vi "Unflatten-JoyButtonEventData.vi"(8 "error in (no error)":errorcluster, 11 "Event Binary Data":string) -> (0 "error out":errorcluster, 3 "Event Data":T1)   [LabVIEW 2026, in "SDL3.lvlib" / "Events.lvlib"]
uses:
  JoyButtonEventData--cluster.ctl
  Joystick/JoystickID--integer.ctl
  Events.lvlib
  Joystick/Joystick.lvlib
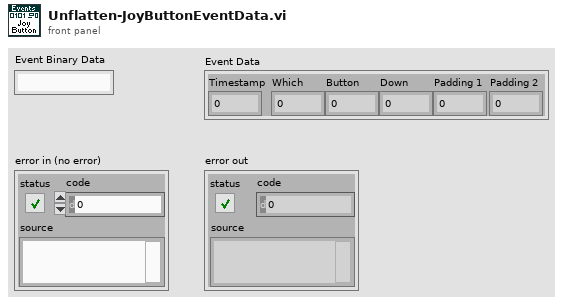
[diagram p1: front panel]
types:
  T1 = typedef "SDL3.lvlib/Events.lvlib/JoyButtonEventData--cluster.ctl" = cluster{"Timestamp":u64, "Which":T2, "Button":u8, "Down":i32, "Padding 1":u8, "Padding 2":u8}
  T2 = typedef "SDL3.lvlib/Joystick.lvlib/JoystickID--integer.ctl" = u32
  T3 = enum16{"big-endian, network order", "native, host order", "little-endian"}
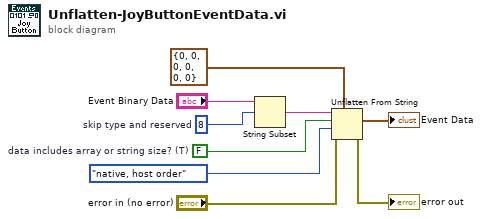
[diagram p0: block diagram]
diagram:
  w3 = 8  # skip type and reserved
  w6 = FALSE  # data includes array or string size? (T)
  n1 = String Subset(string="Event Binary Data", offset (0)=w3) -> (substring=w4:string)  [unwired: 1 in]
  n2 = Unflatten From String(type=T1 {"Timestamp"=0, "Which"=0, "Button"=0, "Down"=0, "Padding 1"=0, "Padding 2"=0} ("JoyButtonEvent"), binary string=w4, data includes array or string size? (T)=w6, byte order (0:big-endian, network order)=T3."native, host order", error in (no error)="error in (no error)") -> (value=→"Event Data":T1, error out=→"error out":errorcluster)  [unwired: 1 out]
